vi "TimeOut.vi"(7 "TimeOut(s)":dbl, 8 "error in":errorcluster, 9 "ElapseTimeIn":u32, 10 "BeforeTime":u32, 11 "CurrentTime":u32) -> (0 "error out":errorcluster, 1 "reset":bool, 2 "ElapseTimeOut":u32, 3 "TimeOut":bool)   [LabVIEW 2015]
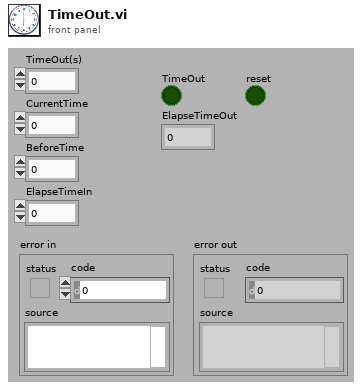
[diagram p1: front panel]
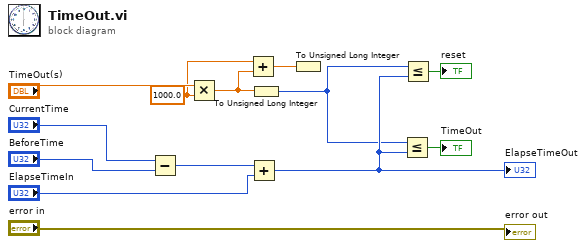
[diagram p0: block diagram]
diagram:
  w2 = 1000.0 ("y")
  n1 = Subtract(x="CurrentTime", y="BeforeTime") -> (x-y=w11:u32)
  n2 = Multiply(x="TimeOut(s)", y=w2) -> (x*y=w3:dbl)
  n3 = Add(x=w2, y=w3) -> (x+y=w4:dbl)
  n4 = Add(x=w11, y="ElapseTimeIn") -> (x+y=w7:u32)
  "ElapseTimeOut" <- w7
  n5 = To Unsigned Long Integer(number=w3) -> (unsigned 32bit integer=w1:u32)
  n6 = To Unsigned Long Integer(number=w4) -> ()  [unwired: 1 out]
  n7 = Less Or Equal?(x=w1, y=w7) -> (x <= y?=→"TimeOut":bool)
  n8 = Less Or Equal?(x=w1, y=w7) -> (x <= y?=→"reset":bool)
  "error out" <- "error in"
